vi "CheckFuncPan.vi"(8 "error in (no error)":errorcluster caption="entrée d'erreur (pas d'erreur)", 9 "Function":string, 10 "LoadedFuncArr":string[](array[string]), 11 "LoadedInst":refnum<class "BaseDevice.lvclass">[](array[class])) -> (0 "error out":errorcluster caption="sortie d'erreur", 1 "PanelName":string="ClassPanel", 2 "OperCanceled":bool, 3 "LoadedInst Out":refnum<class "BaseDevice.lvclass">[](array[class]))   [LabVIEW 2019, in "BaseDevice.lvclass"]
uses:
  BaseDevice.lvclass
  BaseDevice.lvclass/BaseDevice.ctl
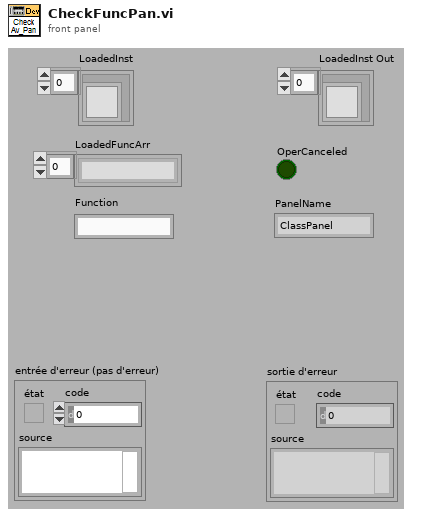
[diagram p1: front panel]
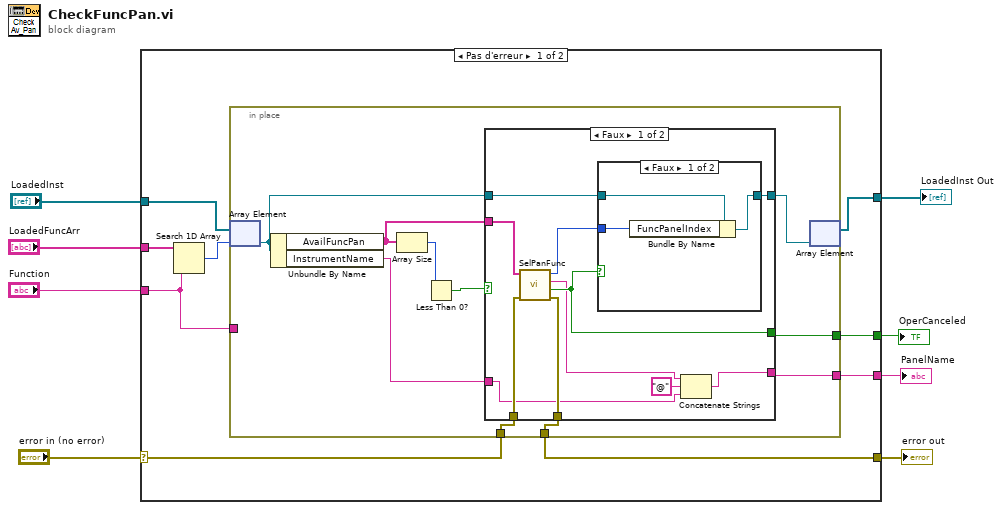
[diagram p0: block diagram]
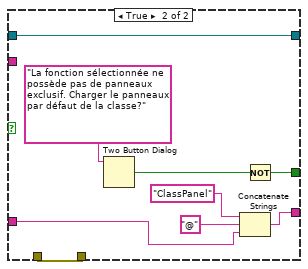
[diagram p3: hidden frame]
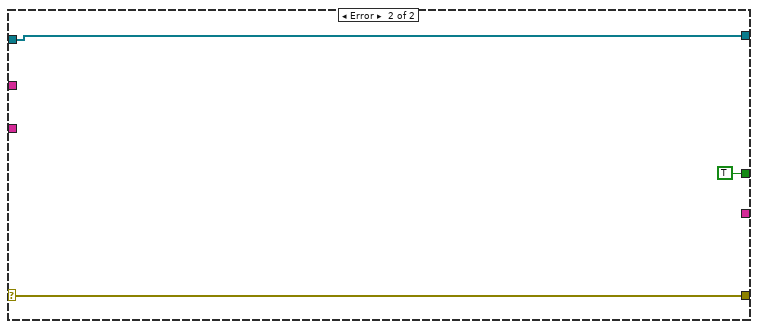
[diagram p4: hidden frame]
diagram:
  n1 = case shown="Pas d'erreur" "error in (no error)" {
    selector: "error in (no error)" -> [w13 w54]
    tunnel: [w12 w54] -> w7
    tunnel: "LoadedInst" -> [w11 w53]
    tunnel: "LoadedFuncArr" -> [w17 _]
    tunnel: "Function" -> [w14 _]
    tunnel: [w16 TRUE ("Canceled")] -> w3
    tunnel: [w15 _] -> w2
    tunnel: [w9 w53] -> w1
    frame No Error {
      n2 = Search 1D Array(1D array=w17, element=w14) -> (index of element=w10:i32)  [unwired: 1 in]
      n3 = in-place {
        in-place-border: [w26] -> w16
        in-place-border: [w25] -> w15
        in-place-border: w14 -> [_]
        in-place-border: w13 -> [w22]
        in-place-border: [w21] -> w12
        n4 = in-place-array #1(w11, w10) -> (w19:refnum<class "BaseDevice.lvclass">)
        n5 = Unbundle By Name(w19) -> ("AvailFuncPan"=w23:string[], "InstrumentName"=w18:string)
        n6 = Array Size(array=w23) -> (size(s)=w24:i32)
        n7 = Less Than 0?(x=w24) -> (x < 0?=w27:bool)
        n8 = case shown="Faux" w27 {
          tunnel: [w35 w47] -> w26
          tunnel: [w30 w48] -> w25
          tunnel: w23 -> [w38 _]
          tunnel: w22 -> [w37 w46]
          tunnel: [w36 w46] -> w21
          tunnel: [w34 w45] -> w20
          tunnel: w19 -> [w33 w45]
          tunnel: w18 -> [w28 w43]
          frame False {
            n9 = call "SelPanFunc.vi"("error in (no error)"=w37, "AvailFunc"=w38) -> ("error out"=w36:errorcluster, "Canceled"=w35:bool, "Selected Panel"=w31:string, "PanelIndex"=w32:i32)  [unwired: 6 in]
            n10 = case shown="Faux" w35 {
              tunnel: [w40 w42] -> w34
              tunnel: w33 -> [w41 w42]
              tunnel: w32 -> [w39 _]
              frame False {
                n11 = Bundle By Name(cluster=w41, "FuncPanelIndex"=w39) -> (w40:refnum<class "BaseDevice.lvclass">)
              }
              frame True {
              }
            }
            n12 = Concatenate Strings(w31, "@" ("chaîne"), w28) -> (w30:string)
          }
          frame True {
            n13 = Two Button Dialog(message="La fonction sélectionnée ne possède pas de panneaux exclusif. Charger le panneaux par défaut de la classe?") -> (T button?=w50:bool)  [unwired: 2 in]
            n14 = Concatenate Strings("ClassPanel" ("message"), "@" ("expression régulière"), w43) -> (w48:string)
            n15 = Not(x=w50) -> (.not. x?=w47:bool)
          }
        }
        n16 = in-place-array #1(w20) -> (w9:refnum<class "BaseDevice.lvclass">[])  [unwired: 1 out]
      }
    }
    frame Error {
    }
  }
  "error out" <- w7
  "OperCanceled" <- w3
  "PanelName" <- w2
  "LoadedInst Out" <- w1
